vi "Initialize Lookup Table - HSYNC.vi"() -> ()   [LabVIEW 2015]
uses:
  <vilib>/measure/NI_MABase.lvlib
panel:
  out "波形图":dbl[](graph)
  out "Init Data Out":i16[](array[numeric])
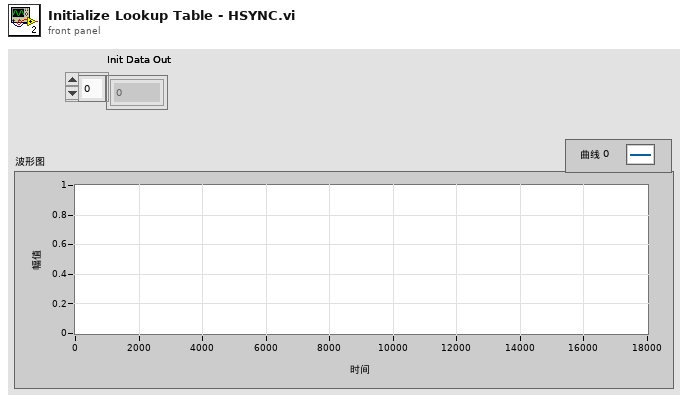
[diagram p1: front panel]
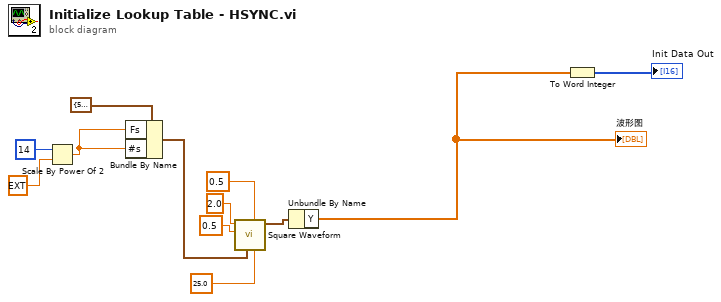
[diagram p0: block diagram]
diagram:
  n1 = Scale By Power Of 2(n=i16 14, x=ext 1.0) -> (x*2^n=w9:ext)
  n2 = Bundle By Name(cluster=cluster{"Fs":dbl, "#s":dbl} {"Fs"=5000.0, "#s"=50.0} ("sampling info"), "Fs"=w9, "#s"=w9) -> (w6:cluster{"Fs":dbl, "#s":dbl})
  n3 = call <vilib>:"Square Waveform.vi"("duty cycle (%)"=25.0, "offset"=0.5, "sampling info"=w6, "amplitude"=0.5, "frequency"=2.0) -> ("signal out"=w5:waveform(dbl))  [unwired: 5 in, 1 out]
  n4 = Unbundle By Name(w5) -> ("Y"=w3:dbl[])
  "波形图" <- w3
  n5 = To Word Integer(number=w3) -> (16bit integer=→"Init Data Out":i16[])
